vi "Discrete Stability Analysis.vi"() -> ()   [LabVIEW 2018]
uses:
  <vilib>/addons/Control Design/_Utility/Rendering.llb/Rendering Transfer Function Options.ctl
  <vilib>/addons/Control Design/_Model Construction/Data Typedefs.llb/CD CtoD Conversion Method.ctl
  <vilib>/addons/Control Design/_Model Construction/Model Typedefs.llb/CD Transfer Function Model (MIMO).ctl
  <vilib>/addons/Control Design/_Model Construction/Model Typedefs.llb/CD General Elements.ctl
  <vilib>/addons/Control Design/_Model Construction/Model Typedefs.llb/CD Transfer Function Model (SISO).ctl
  <vilib>/addons/Control Design/_Model Conversions/Continuous and Discrete.llb/Continuous and Discrete SubVI/cd_Convert Continuous to Discrete (TF).vi
  <vilib>/addons/Control Design/_Utility/Model Viewer.llb/Model Viewer SubVI/cd_Draw Transfer Function Equation (TF).vi
  <vilib>/addons/Control Design/_Dynamic Analysis/Dynamic Analysis.llb/Dynamic Analysis subVI/cd_Root Locus (Transfer Function).vi
  <vilib>/addons/Control Design/_Model Interconnection/Model Interconnection.llb/Model Interconnection SubVI/cd_Unit Feedback (TF and TF).vi
  <vilib>/addons/Control Design/_Time Response Analysis/Time Response.llb/Time Response subVI/cd_Step Response (Transfer Function).vi
  <vilib>/addons/Control Design/_Model Interconnection/Model Interconnection.llb/Model Interconnection SubVI/cd_Matrix Multiply Models (TF and TF).vi
  <vilib>/addons/Control Design/_Frequency Response Analysis/Frequency Response.llb/Frequency Response subVI/cd_Gain and Phase Margin (Transfer Function).vi
  <vilib>/addons/Control Design/_Model Construction/NI_LinSys_Model Typedefs.lvlib
  <vilib>/addons/Control Design/_Utility/NI_CD_Model Viewer.lvlib
  <vilib>/addons/Control Design/_Utility/NI_LinSys_Rendering.lvlib
  <vilib>/addons/Control Design/_Dynamic Analysis/NI_CD_Dynamic Analysis.lvlib
  <vilib>/addons/Control Design/_Model Conversions/NI_CD_Continuous and Discrete.lvlib
  <vilib>/addons/Control Design/_Time Response Analysis/NI_CD_Time Response.lvlib
  <vilib>/addons/Control Design/_Model Construction/NI_LinSys_Data Typedefs.lvlib
  <vilib>/addons/Control Design/_Model Interconnection/NI_CD_Model Interconnection.lvlib
  <vilib>/addons/Control Design/_Frequency Response Analysis/NI_CD_Frequency Response.lvlib
panel:
  out "Phase Plot":cluster{"W":dbl[], "Phase":dbl[]}[](graph)
  out "Magnitude Plot":cluster{"W":dbl[], "Magnitude":dbl[]}[](graph)
  in  "C":dbl=1.0 format="%#_13g"
  in  "K":dbl=1.0
  out "Closed-loop Step Response":cluster{"time":dbl[], dbl[]}[](graph)
  in  "tau":dbl=1.0 format="%#_13g"
  in  "Sampling period (s)":dbl=1.0 format="%#_13g"
  out "Root Locus Plot":cluster{"W":dbl[], "Magnitude":dbl[]}[](graph)
  out "G_p(z)":picture
  # "Controls Board"
  # "Discrete Stability Analysis"
  # "Plant"
  # "Controller"
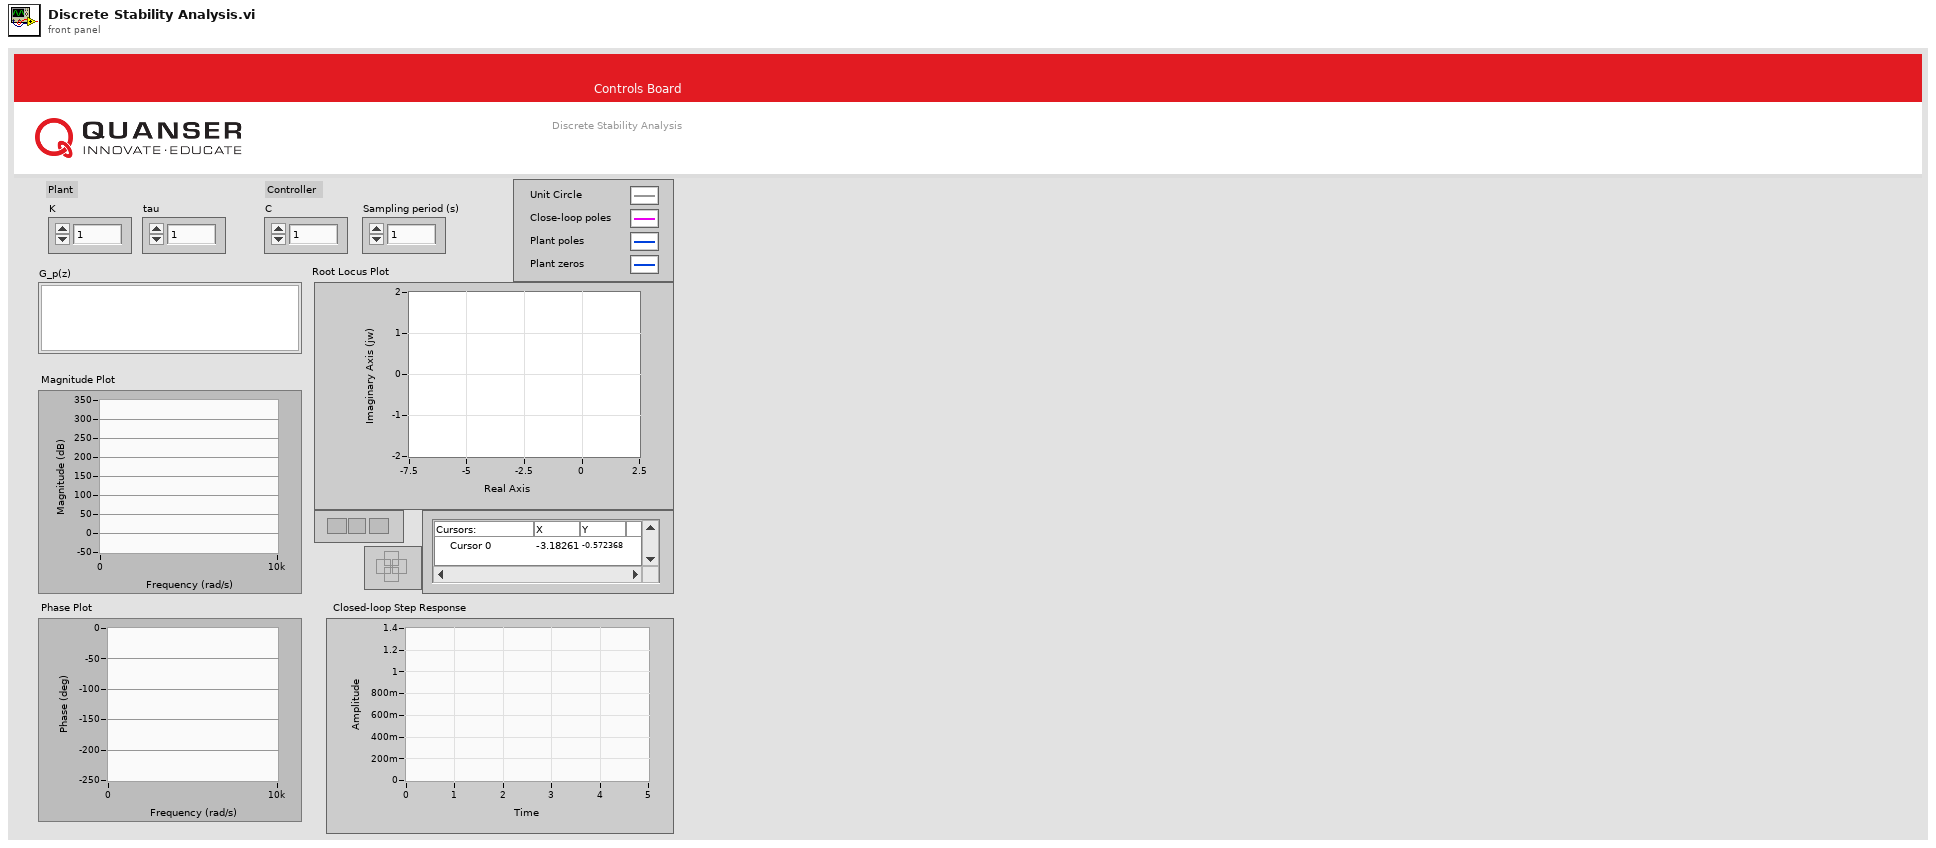
[diagram p1: front panel]
types:
  T1 = typedef "NI_LinSys_Model Typedefs.lvlib/CD General Elements.ctl" = cluster{"Model name":string, "Input names":string[], "Output names":string[], "Input Delays":dbl[], "Output Delays":dbl[], "Sampling Time":dbl, "Notes":string}
  T2 = typedef "NI_LinSys_Model Typedefs.lvlib/CD Transfer Function Model (MIMO).ctl" = cluster{"properties":T1, "transfer function(s)":T3[][]}
  T3 = typedef "NI_LinSys_Model Typedefs.lvlib/CD Transfer Function Model (SISO).ctl" = cluster{"Numerator":dbl[], "Denominator":dbl[], "delay":dbl}
  T4 = typedef "NI_LinSys_Data Typedefs.lvlib/CD CtoD Conversion Method.ctl" = u16
  T5 = typedef "NI_LinSys_Rendering.lvlib/Rendering Transfer Function Options.ctl" = u16
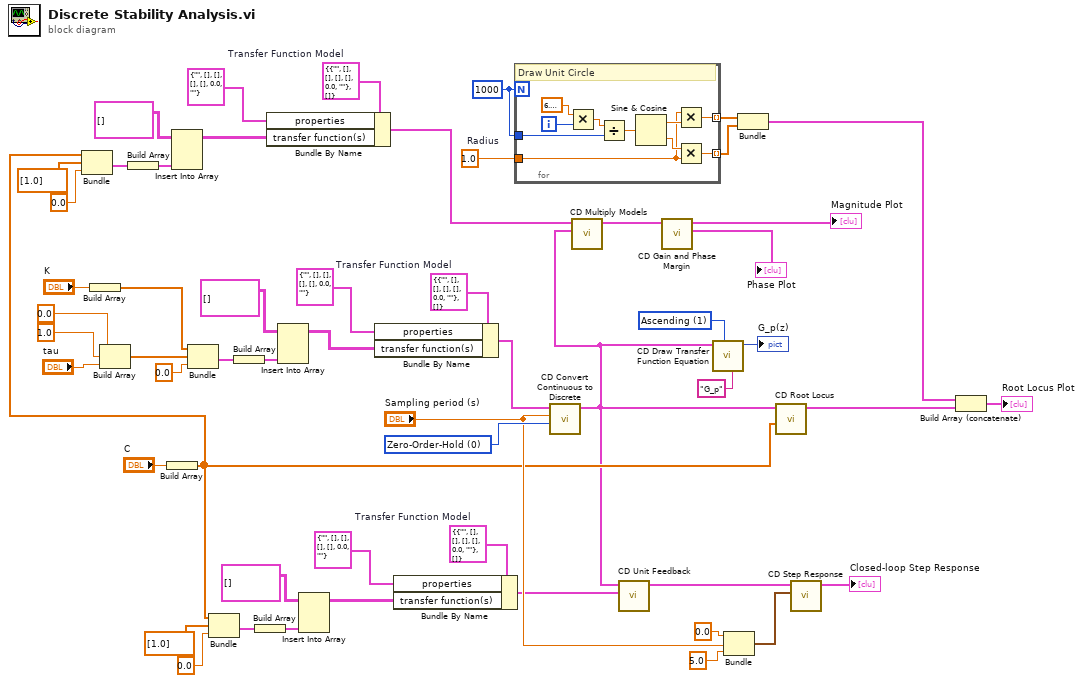
[diagram p0: block diagram]
diagram:
  w7 = T2 {"properties"={"Model name"="", "Input names"=[], "Output names"=[], "Input Delays"=[], "Output Delays"=[], "Sampling Time"=0.0, "Notes"=""}, "transfer function(s)"=[]}  # Transfer Function Model
  w38 = T2 {"properties"={"Model name"="", "Input names"=[], "Output names"=[], "Input Delays"=[], "Output Delays"=[], "Sampling Time"=0.0, "Notes"=""}, "transfer function(s)"=[]}  # Transfer Function Model
  w54 = T2 {"properties"={"Model name"="", "Input names"=[], "Output names"=[], "Input Delays"=[], "Output Delays"=[], "Sampling Time"=0.0, "Notes"=""}, "transfer function(s)"=[]}  # Transfer Function Model
  w45 = T4 0 items=["Zero-Order-Hold", "Tustin (Bilinear)", "Prewarp", "Forward", "Backward", "Z-Transform", "First-Order-Hold", "Matched Pole-Zero"] ("Method")
  w48 = T5 1 items=["Descending", "Ascending", "Negative Power"] ("Display Format")
  w50 = 1.0  # Radius
  w53 = 1000
  n1 = Build Array("K") -> (w19:dbl[])
  n2 = Build Array(0.0, 1.0, "tau") -> (w23:dbl[])
  n3 = Build Array("C") -> (w6:dbl[])
  n4 = Bundle(w6, dbl[] [1.0], 0.0) -> (w12:cluster{dbl[], dbl[], dbl})  [unwired: 1 in]
  n5 = Build Array(w12) -> (w14:cluster{dbl[], dbl[], dbl}[])
  n6 = Insert Into Array(array=cluster{dbl[], dbl[], dbl}[][] [], new element=w14) -> (w13:cluster{dbl[], dbl[], dbl}[][])  [unwired: 2 in]
  n7 = Bundle(w19, w23, 0.0) -> (w29:cluster{dbl[], dbl[], dbl})  [unwired: 1 in]
  n8 = Bundle(w6, dbl[] [1.0], 0.0) -> (w32:cluster{dbl[], dbl[], dbl})  [unwired: 1 in]
  n9 = Build Array(w29) -> (w22:cluster{dbl[], dbl[], dbl}[])
  n10 = Build Array(w32) -> (w31:cluster{dbl[], dbl[], dbl}[])
  n11 = Bundle By Name(cluster=w7, "properties"=T1 {"Model name"="", "Input names"=[], "Output names"=[], "Input Delays"=[], "Output Delays"=[], "Sampling Time"=0.0, "Notes"=""}, "transfer function(s)"=w13) -> (w4:T2)
  n12 = Insert Into Array(array=cluster{dbl[], dbl[], dbl}[][] [], new element=w22) -> (w21:cluster{dbl[], dbl[], dbl}[][])  [unwired: 2 in]
  n13 = Insert Into Array(array=cluster{dbl[], dbl[], dbl}[][] [], new element=w31) -> (w30:cluster{dbl[], dbl[], dbl}[][])  [unwired: 2 in]
  n14 = Bundle By Name(cluster=w54, "properties"=T1 {"Model name"="", "Input names"=[], "Output names"=[], "Input Delays"=[], "Output Delays"=[], "Sampling Time"=0.0, "Notes"=""}, "transfer function(s)"=w21) -> (w39:T2)
  n15 = Bundle By Name(cluster=w38, "properties"=T1 {"Model name"="", "Input names"=[], "Output names"=[], "Input Delays"=[], "Output Delays"=[], "Sampling Time"=0.0, "Notes"=""}, "transfer function(s)"=w30) -> (w36:T2)
  n16 = for {
    N: w53 -> [_]
    tunnel: w53 -> [w63]
    tunnel: [w57] -> w52 mode=indexing
    tunnel: [w56] -> w51 mode=indexing
    tunnel: w50 -> [w58]
    i -> [w61]
    # "Draw Unit Circle"
    n17 = Multiply(x=6.283185307179586, y=w61) -> (x*y=w65:dbl)
    n18 = Divide(x=w65, y=w63) -> (x/y=w64:dbl)
    n19 = Sine & Cosine(0:w64) -> (1:w60:dbl, 2:w59:dbl)
    n20 = Multiply(x=w58, y=w60) -> (x*y=w57:dbl)
    n21 = Multiply(x=w59, y=w58) -> (x*y=w56:dbl)
  }
  n22 = call-poly <vilib>:"CD Convert Continuous to Discrete.vi"("Method"=w45, "Sampling Time (s)"="Sampling period (s)", "Continuous Transfer Function Model"=w39) -> ("Discrete Transfer Function Model"=w5:T2)  [unwired: 7 in, 1 out]
  n23 = call-poly <vilib>:"CD Multiply Models.vi"("Model 2"=w5, "Model 1"=w4) -> ("Model Out"=w3:T2)  [unwired: 8 in, 1 out]
  n24 = call-poly <vilib>:"CD Unit Feedback.vi"("Model 2"=w36, "Model 1"=w5) -> ("Closed-Loop Model"=w18:T2)  [unwired: 8 in, 1 out]
  n25 = call-poly <vilib>:"CD Gain and Phase Margin.vi"("Transfer Function Model"=w3) -> ("Phase Plot"=→"Phase Plot":cluster{"W":dbl[], "Phase":dbl[]}[], "Magnitude Plot"=→"Magnitude Plot":cluster{"W":dbl[], "Magnitude":dbl[]}[])  [unwired: 6 in, 3 out]
  n26 = call-poly <vilib>:"CD Draw Transfer Function Equation.vi"("Function Name (empty)"="G_p", "Display Format"=w48, "Transfer Function Model"=w5) -> ("Equation"=→"G_p(z)":picture)  [unwired: 6 in, 2 out]
  n27 = Bundle(0.0, "Sampling period (s)"="Sampling period (s)", 5.0) -> (w40:cluster{dbl, "Sampling period (s)":dbl, dbl})  [unwired: 1 in]
  n28 = Bundle(w52, w51) -> (w17:cluster{dbl[], dbl[]})  [unwired: 1 in]
  n29 = call-poly <vilib>:"CD Root Locus.vi"("Gain"=w6, "Transfer Function Model"=w5) -> ("Root Locus Graph"=w16:cluster{dbl[], dbl[]}[])  [unwired: 6 in, 3 out]
  n30 = call-poly <vilib>:"CD Step Response.vi"("Time Range"=w40, "Transfer Function Model"=w18) -> ("Step Response Graph"=→"Closed-loop Step Response":cluster{"time":dbl[], dbl[]}[])  [unwired: 7 in, 2 out]
  n31 = Build Array (concatenate)(w17, w16) -> (→"Root Locus Plot":cluster{dbl[], dbl[]}[])
